vi "Get Alarm 1 Hi.vi"(8 "error in":errorcluster, 11 "Cfg Dev in":refnum<class "CnPt.lvclass">) -> (0 "error out":errorcluster, 2 "Alarm 2 Hi":dbl, 3 "Cfg Dev out":refnum<class "CnPt.lvclass">)   [LabVIEW 2015, in "CnPt.lvclass"]
uses:
  CnPt.lvclass
  <vilib>/MSR Consulting, LLC/General Reuse/Session APIs/Serial/Serial Session.lvclass
  CnPt.lvclass/CnPt.ctl
  <vilib>/MSR Consulting, LLC/General Reuse/Session APIs/Serial/Public/Asynchronous Write.vi
  <vilib>/MSR Consulting, LLC/General Reuse/Session APIs/Serial/Public/Asynchronous Read.vi
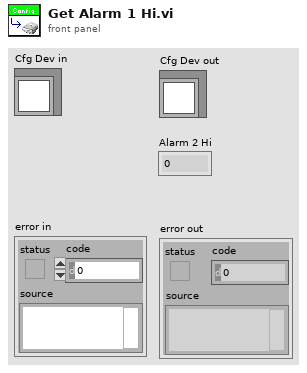
[diagram p1: front panel]
types:
  T1 = typedef "Serial Session.lvclass/Session Handle.ctl" = refnum<data-value>
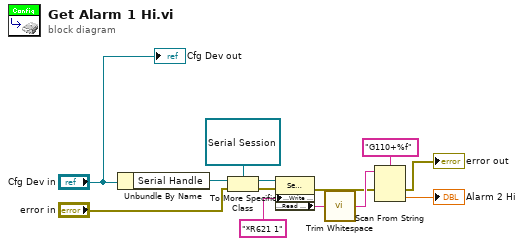
[diagram p0: block diagram]
diagram:
  n1 = Unbundle By Name("Cfg Dev in") -> ("Serial Handle"=w13:T1)
  n2 = To More Specific Class(target class=refnum<data-value> refnum, reference=w13, error in="error in") -> (specific class reference=w11:refnum<data-value>, error out=w9:errorcluster)
  n3 = property class="Serial Session"(reference=w11, error in=w9, "Public:Write - Asynchronous"="*R621 1" ("format string")) -> (error out=w3:errorcluster, "Public:Read - Asynchronous"=w5:string)  [unwired: 1 out]
  n4 = call <vilib>:"Trim Whitespace.vi"("string"=w5) -> ("trimmed string"=w4:string)  [unwired: 1 in]
  n5 = Scan From String(format string="G110+%f", input string=w4, error in=w3) -> (error out=→"error out":errorcluster, output 1=→"Alarm 2 Hi":dbl)  [unwired: 2 in, 2 out]
  "Cfg Dev out" <- "Cfg Dev in"
